vi "a.F.b.u.s.A bearbeiten.vi"(8 "error in (no error)":errorcluster caption="Fehler (Eingang, kein Fehler)", 9 "Farbwerte":T1={"Rot-min."=230.0, "Rot.max."=240.0, "Blau-min."=300.0, "Blau-max."=320.0, "Grün-min."=312.0, "Grün-max."=319.0, "Weiß-min."=220.0, "Weiß-max."=230.0}, 10 "Stop?":bool, 11 "Device ID":T2(ring)) -> (0 "error out":errorcluster caption="Fehler (Ausgang)", 2 "fehlbarbeitung?":bool, 3 "Device ID Out":T2(ring))   [LabVIEW 2010]
uses:
  sub VIs v Hauptprogramm/globale Variable 1.vi
panel:
  out "Numerisches Element":i32
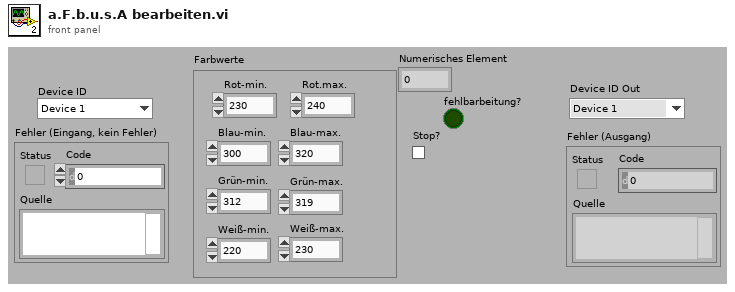
[diagram p1: front panel]
types:
  T1 = cluster{"Rot-min.":dbl, "Rot.max.":dbl, "Blau-min.":dbl, "Blau-max.":dbl, "Grün-min.":dbl, "Grün-max.":dbl, "Weiß-min.":dbl, "Weiß-max.":dbl}
  T2 = enum16{"Device 1", "Device 2", "Device 3", "Device 4", "Device 5", "Device 6", "Device 7", "Device 8"}
  T3 = enum8{"Power 1", "Power 2", "Power 3", "Power 4", "Power 5", "Power 6", "Power 7", "Power 8"}
  T4 = enum8{"Output 1 (O1)", "Output 2 (O2)", "Output 3 (O3)", "Output 4 (O4)", "Output 5 (O5)", "Output 6 (O6)", "Output 7 (O7)", "Output 8 (O8)"}
  T5 = enum8{"Robo Interface", "Extension 1", "Extension 2", "Extension 3"}
  T6 = enum16{"Left Button", "Center Button", "Right Button", "Window Close"}
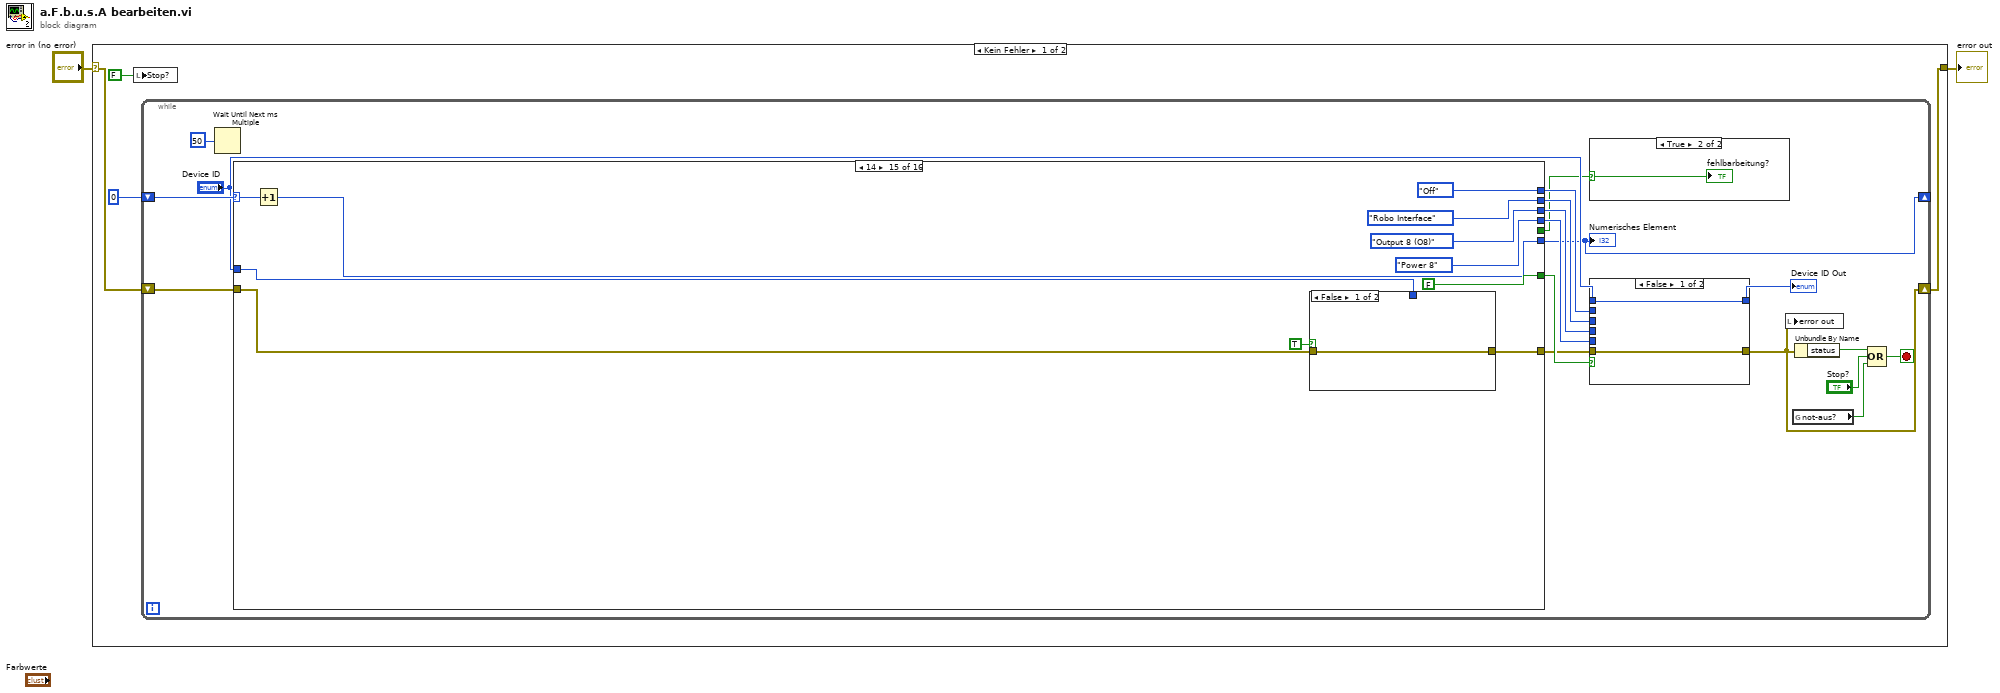
[diagram p0: block diagram]
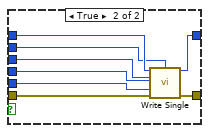
[diagram p3: hidden frame]
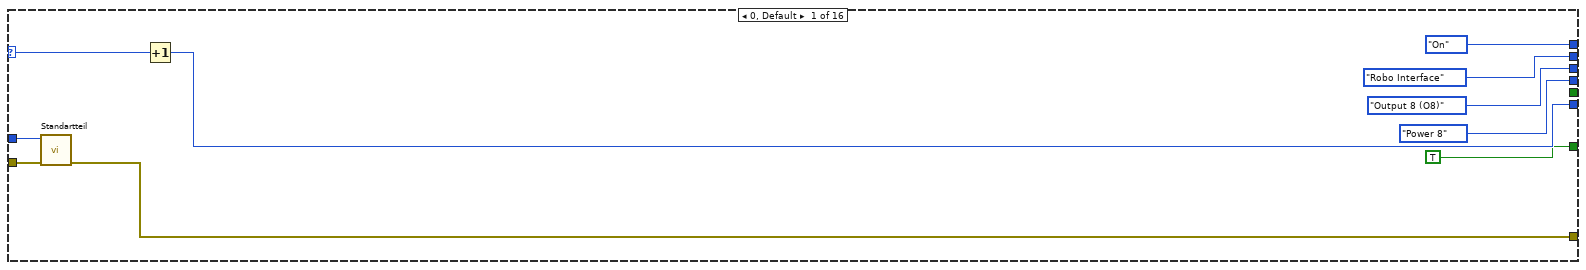
[diagram p4: hidden frame]
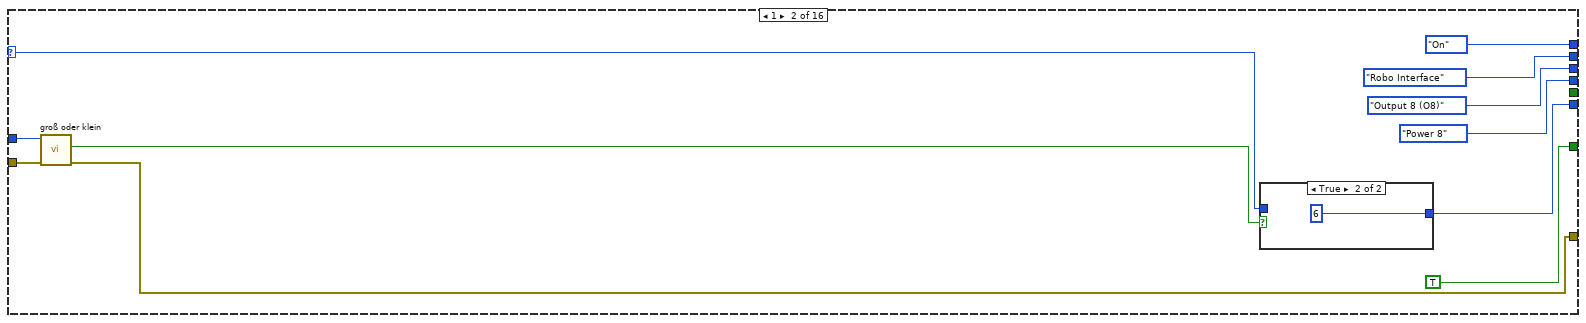
[diagram p5: hidden frame]
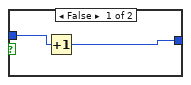
[diagram p6: hidden frame]
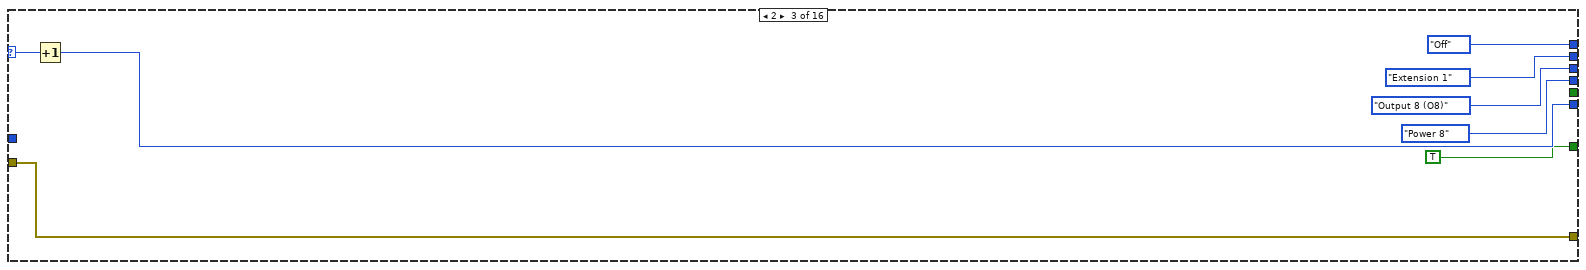
[diagram p7: hidden frame]
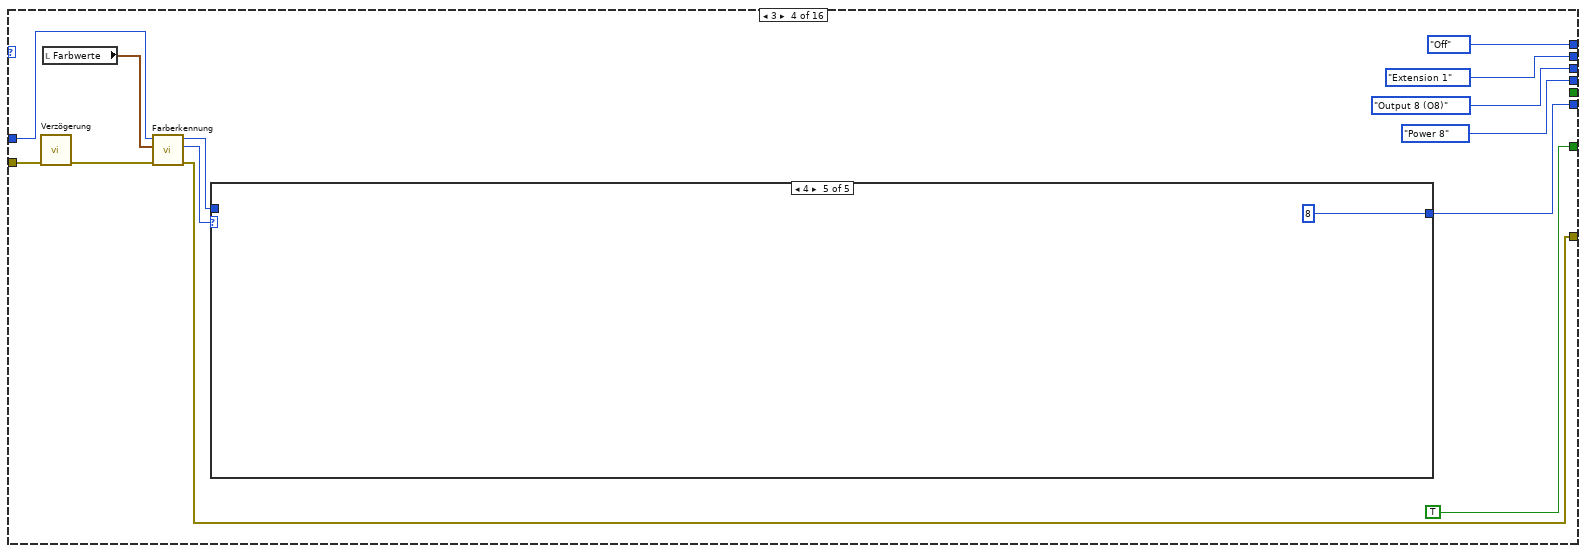
[diagram p8: hidden frame]
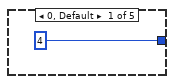
[diagram p9: hidden frame]
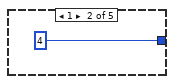
[diagram p10: hidden frame]
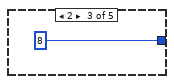
[diagram p11: hidden frame]
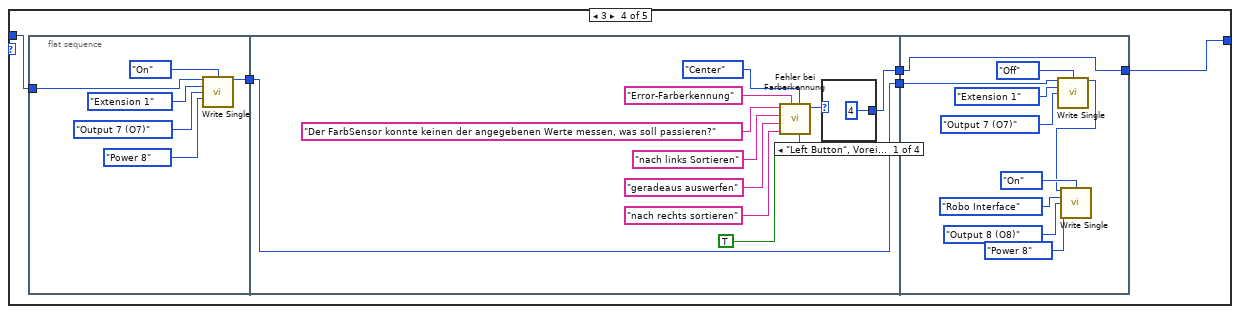
[diagram p12: hidden frame]
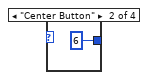
[diagram p13: hidden frame]
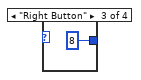
[diagram p14: hidden frame]
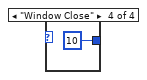
[diagram p15: hidden frame]
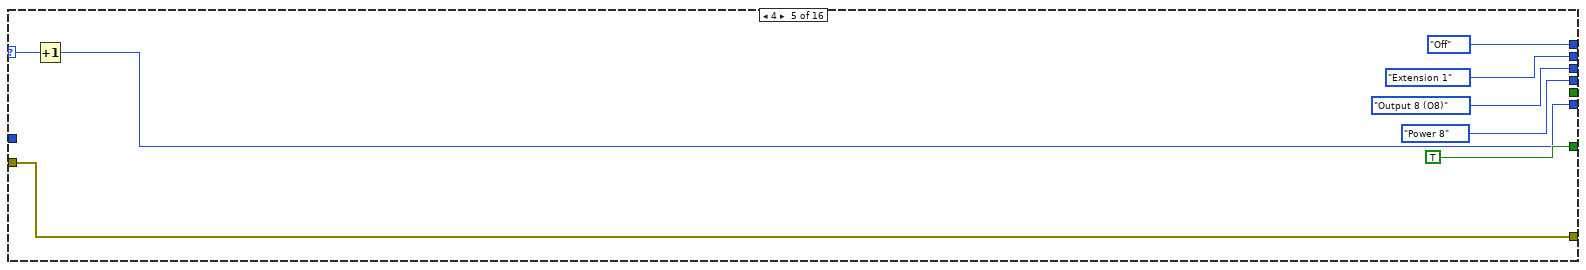
[diagram p16: hidden frame]
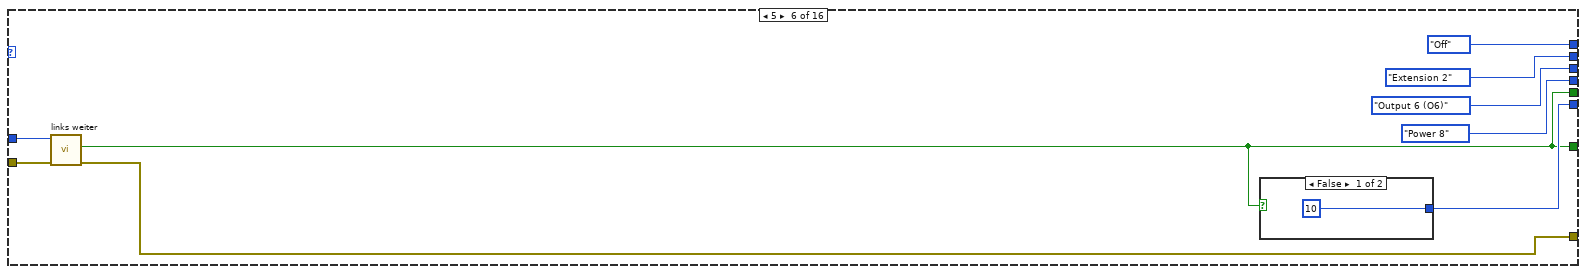
[diagram p17: hidden frame]
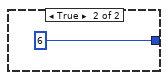
[diagram p18: hidden frame]
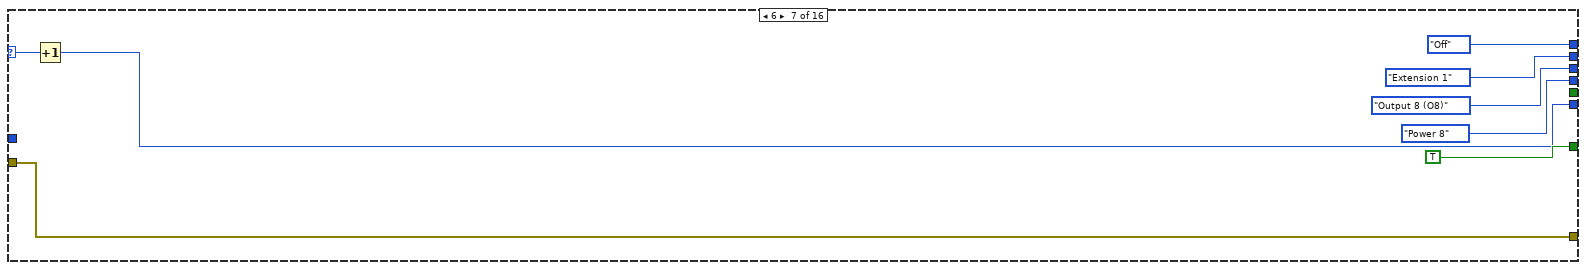
[diagram p19: hidden frame]
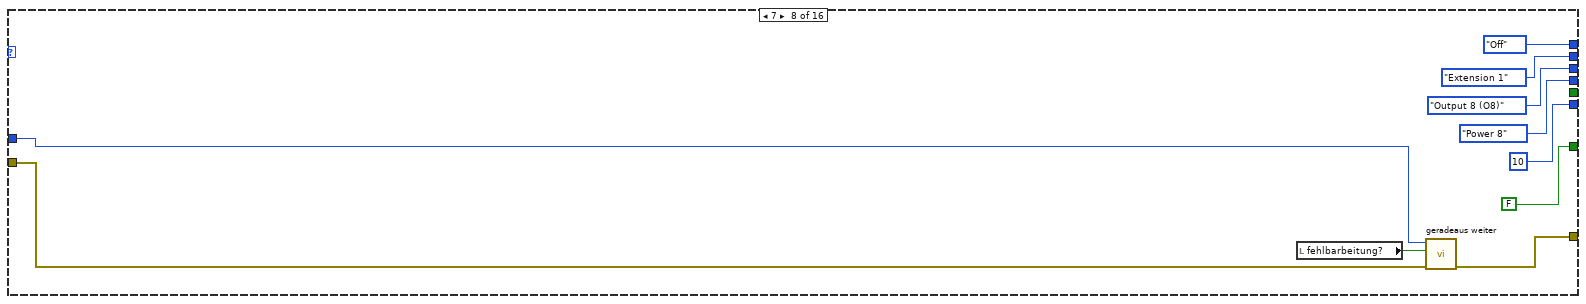
[diagram p20: hidden frame]
diagram:
  n1 = case shown="Kein Fehler" "error in (no error)" {
    selector: "error in (no error)" -> [w4 w233]
    tunnel: [w5 w233] -> w1
    frame No Error {
      n2 = local write "Stop?"(FALSE ("Stop?")) -> ()
      n3 = while {
        shift-right: [w7] -> _
        shift-left: 0 -> [w12]
        shift-right: [w16] -> w5
        shift-left: w4 -> [w9]
        stop <- w13 stop-if-true
        n4 = Wait Until Next ms Multiple(millisecond multiple=50) -> ()  [unwired: 1 out]
        n5 = case shown="14" w12 {
          selector: w12 -> [w36 w46 w66 _ w122 _ w140 _ w158 _ w177 w185 w193 w201 w213 w226]
          tunnel: [w45 w47 w67 w72 w120 w129 w141 10 w159 w167 w178 w186 w194 w200 w212 w226] -> w7
          tunnel: [T3."Power 8" ("Output_PWM") T3."Power 8" ("Output_PWM") T3."Power 8" ("Output_PWM") T3."Power 8" ("Output_PWM") T3."Power 8" ("Output_PWM") T3."Power 8" ("Output_PWM") T3."Power 8" ("Output_PWM") T3."Power 8" ("Output_PWM") T3."Power 8" ("Output_PWM") T3."Power 8" ("Output_PWM") T3."Power 8" ("Output_PWM") T3."Power 8" ("Output_PWM") T3."Power 8" ("Output_PWM") T3."Power 8" ("Output_PWM") T3."Power 8" ("Output_PWM") T3."Power 8" ("Output_PWM")] -> w23
          tunnel: [T5."Robo Interface" ("Module") T5."Robo Interface" ("Module") T5."Extension 1" ("Module") T5."Extension 1" ("Module") T5."Extension 1" ("Module") T5."Extension 2" ("Module") T5."Extension 1" ("Module") T5."Extension 1" ("Module") T5."Extension 1" ("Module") T5."Extension 2" ("Module") T5."Extension 1" ("Module") T5."Extension 1" ("Module") T5."Extension 1" ("Module") T5."Robo Interface" ("Module") T5."Robo Interface" ("Module") T5."Robo Interface" ("Module")] -> w22
          tunnel: [T4."Output 8 (O8)" ("Single_Output") T4."Output 8 (O8)" ("Single_Output") T4."Output 8 (O8)" ("Single_Output") T4."Output 8 (O8)" ("Single_Output") T4."Output 8 (O8)" ("Single_Output") T4."Output 6 (O6)" ("Single_Output") T4."Output 8 (O8)" ("Single_Output") T4."Output 8 (O8)" ("Single_Output") T4."Output 8 (O8)" ("Single_Output") T4."Output 7 (O7)" ("Single_Output") T4."Output 1 (O1)" ("Single_Output") T4."Output 2 (O2)" ("Single_Output") T4."Output 3 (O3)" ("Single_Output") T4."Output 8 (O8)" ("Single_Output") T4."Output 8 (O8)" ("Single_Output") T4."Output 8 (O8)" ("Single_Output")] -> w21
          tunnel: [enum8{"Off", "On"}."On" ("Output_Action") enum8{"Off", "On"}."On" ("Output_Action") enum8{"Off", "On"}."Off" ("Output_Action") enum8{"Off", "On"}."Off" ("Output_Action") enum8{"Off", "On"}."Off" ("Output_Action") enum8{"Off", "On"}."Off" ("Output_Action") enum8{"Off", "On"}."Off" ("Output_Action") enum8{"Off", "On"}."Off" ("Output_Action") enum8{"Off", "On"}."Off" ("Output_Action") enum8{"Off", "On"}."Off" ("Output_Action") enum8{"Off", "On"}."Off" ("Output_Action") enum8{"Off", "On"}."On" ("Output_Action") enum8{"Off", "On"}."On" ("Output_Action") enum8{"Off", "On"}."Off" ("Output_Action") enum8{"Off", "On"}."Off" ("Output_Action") enum8{"Off", "On"}."Off" ("Output_Action")] -> w20
          tunnel: [w39 w49 w60 w74 w121 w130 w139 w149 w157 w168 w176 w184 w192 w202 w209 w227] -> w17
          tunnel: w9 -> [w38 w50 w60 w69 w121 w132 w139 w150 w157 w169 w176 w184 w192 w202 w210 w227]
          tunnel: [TRUE ("AN/Aus") TRUE ("AN/Aus") TRUE ("AN/Aus") TRUE ("AN/Aus") TRUE ("AN/Aus") w128 TRUE ("AN/Aus") FALSE ("AN/Aus") TRUE ("AN/Aus") w165 TRUE ("AN/Aus") TRUE ("AN/Aus") TRUE ("AN/Aus") TRUE ("AN/Aus") FALSE ("AN/Aus") FALSE ("AN/Aus")] -> w18
          tunnel: "Device ID" -> [w37 w51 _ w71 _ w131 _ w151 _ w166 _ _ _ _ w211 _]
          tunnel: [_ _ _ _ _ w128 _ _ _ w165 _ _ _ _ _ _] -> w8
          frame 0, Default {
            n6 = call "Standartteil.vi"("error in (no error)"=w38, "Device ID"=w37) -> ("error out"=w39:errorcluster)  [unwired: 8 out]
            n7 = Increment(x=w36) -> (x+1=w45:i32)
          }
          frame 1 {
            n8 = call "groß oder klein.vi"("error in (no error)"=w50, "Device ID"=w51) -> ("error out"=w49:errorcluster, "Groß?"=w48:bool)  [unwired: 8 out]
            n9 = case shown="True" w48 {
              tunnel: [w58 6] -> w47
              tunnel: w46 -> [w57 _]
              frame False {
                n10 = Increment(x=w57) -> (x+1=w58:i32)
              }
              frame True {
              }
            }
          }
          frame 2 {
            n11 = Increment(x=w66) -> (x+1=w67:i32)
          }
          frame 3 {
            n12 = call "Verzögerung"("error in (no error)"=w69) -> ("error out"=w70:errorcluster)  [unwired: 1 in, 9 out]
            n13 = local read "Farbwerte"() -> (w75:T1)
            n14 = call "Farberkennung.vi"("error in (no error)"=w70, "Farbwerte"=w75, "Device ID"=w71) -> ("error out"=w74:errorcluster, "Farbe"=w73:u16, "Device ID Out"=w68:T2)  [unwired: 2 in, 4 out]
            n15 = case shown="4" w73 {
              tunnel: [4 4 8 w88 8] -> w72
              tunnel: w68 -> [_ _ _ w86 _]
              frame 0, Default {
              }
              frame 1 {
              }
              frame 2 {
              }
              frame 3 {
                n16 = flat-sequence {
                  tunnel: w86 -> [w94]
                  tunnel: [w89] -> w84
                  tunnel: [w98] -> w87
                  tunnel: [w95] -> w85
                  tunnel: w84 -> [w95]
                  tunnel: [w118] -> w88
                  tunnel: w87 -> [w118]
                  tunnel: w85 -> [w117]
                  frame #0 {
                    n17 = call "Write Single.vi"("Device ID"=w94, "Output_Action"=enum8{"Off", "On"}."On", "Module"=T5."Extension 1", "Single_Output"=T4."Output 7 (O7)", "Output_PWM"=T3."Power 8") -> ("Device ID Out"=w89:T2)  [unwired: 1 in, 9 out]
                  }
                  frame #1 {
                    n18 = call "Fehler bei Farberkennung.vi"("Allow user to close window? (TRUE)"=TRUE, "Justify Message (Left)"=enum16{"Left", "Center", "Right"}."Center", "Window Title (\"\")"="Error-Farberkennung" ("Window Title (\"\")"), "Right Button Text (\"Cancel\")"="nach rechts sortieren" ("Center Button Text (\"No\")"), "Center Button Text (\"No\")"="geradeaus auswerfen" ("Right Button Text (\"Cancel\")"), "Left Button Text (\"Yes\")"="nach links Sortieren" ("Left Button Text (\"Yes\")"), "message"="Der FarbSensor konnte keinen der angegebenen Werte messen, was soll passieren?") -> ("Which Button?"=w99:T6)  [unwired: 4 out]
                    n19 = case shown="\"Left Button\", Voreinstellung" w99 {
                      tunnel: [4 6 8 10] -> w98
                      frame "Left Button", Default {
                      }
                      frame "Center Button" {
                      }
                      frame "Right Button" {
                      }
                      frame "Window Close" {
                      }
                    }
                  }
                  frame #2 {
                    n20 = call "Write Single.vi"("Device ID"=w117, "Output_Action"=enum8{"Off", "On"}."Off", "Module"=T5."Extension 1", "Single_Output"=T4."Output 7 (O7)") -> ("Device ID Out"=w110:T2)  [unwired: 2 in, 9 out]
                    n21 = call "Write Single.vi"("Device ID"=w110, "Output_Action"=enum8{"Off", "On"}."On", "Module"=T5."Robo Interface", "Single_Output"=T4."Output 8 (O8)", "Output_PWM"=T3."Power 8") -> ()  [unwired: 1 in, 10 out]
                  }
                }
              }
              frame 4 {
              }
            }
          }
          frame 4 {
            n22 = Increment(x=w122) -> (x+1=w120:i32)
          }
          frame 5 {
            n23 = call "links weiter.vi"("error in (no error)"=w132, "Device ID"=w131) -> ("error out"=w130:errorcluster, "geradeaus?"=w128:bool)  [unwired: 8 out]
            n24 = case shown="False" w128 {
              tunnel: [10 6] -> w129
              frame False {
              }
              frame True {
              }
            }
          }
          frame 6 {
            n25 = Increment(x=w140) -> (x+1=w141:i32)
          }
          frame 7 {
            n26 = local read "fehlbarbeitung?"() -> (w147:bool)
            n27 = call "geradeaus weiter.vi"("error in (no error)"=w150, "fehlbearbeitung?"=w147, "Device ID"=w151) -> ("error out"=w149:errorcluster)  [unwired: 8 out]
          }
          frame 8 {
            n28 = Increment(x=w158) -> (x+1=w159:i32)
          }
          frame 9 {
            n29 = call "rechst weiter.vi"("error in (no error)"=w169, "Device ID"=w166) -> ("error out"=w168:errorcluster, "geradeaus?"=w165:bool)  [unwired: 8 out]
            n30 = case shown="False" w165 {
              tunnel: [10 6] -> w167
              frame False {
              }
              frame True {
              }
            }
          }
          frame 10 {
            n31 = Increment(x=w177) -> (x+1=w178:i32)
          }
          frame 11 {
            n32 = Increment(x=w185) -> (x+1=w186:i32)
          }
          frame 12 {
            n33 = Increment(x=w193) -> (x+1=w194:i32)
          }
          frame 13 {
            n34 = Increment(x=w201) -> (x+1=w200:i32)
          }
          frame 14 {
            n35 = Increment(x=w213) -> (x+1=w212:i32)
            n36 = case shown="False" TRUE {
              tunnel: w211 -> [_ w224]
              tunnel: w210 -> [w219 w221]
              tunnel: [w219 w220] -> w209
              frame False {
              }
              frame True {
                n37 = call "Pneumatik.vi"("error in (no error)"=w221, "Single_Output"=T4."Output 1 (O1)", "Module"=T5."Extension 3", "Device ID"=w224) -> ("error out"=w220:errorcluster)  [unwired: 7 out]
              }
            }
          }
          frame 15 {
            n38 = local write "Stop?"(TRUE) -> ()
          }
        }
        "Numerisches Element" <- w7
        n39 = case shown="True" w8 {
          selector: w8 -> [_ w25]
          frame False {
          }
          frame True {
            "fehlbarbeitung?" <- w25
          }
        }
        n40 = case shown="False" w18 {
          tunnel: "Device ID" -> [w27 w35]
          tunnel: [w27 w34] -> w24
          tunnel: [w26 w33] -> w16
          tunnel: w23 -> [_ w32]
          tunnel: w22 -> [_ w31]
          tunnel: w21 -> [_ w30]
          tunnel: w20 -> [_ w29]
          tunnel: w17 -> [w26 w28]
          frame False {
          }
          frame True {
            n41 = call "Write Single.vi"("Device ID"=w35, "Output_Action"=w29, "Module"=w31, "Single_Output"=w30, "Output_PWM"=w32, "error in"=w28) -> ("Device ID Out"=w34:T2, "error out"=w33:errorcluster)  [unwired: 8 out]
          }
        }
        "Device ID Out" <- w24
        n42 = local write "error out"(w16) -> ()
        n43 = global read "globale Variable 1.vi" "not-aus?"() -> (w10:bool)
        n44 = Unbundle By Name(w16) -> ("status"=w15:bool)
        n45 = Compound Arithmetic op=OR(w15, "Stop?", w10) -> (w13:bool)
      }
    }
    frame Error {
    }
  }
  "error out" <- w1
